vi "Function_Light.vi"(7 "Light Action":T1, 8 "Error in":errorcluster, 10 "Intensity":u8, 11 "Channel":u8) -> (0 "Error Out":errorcluster)   [LabVIEW 2013]
uses:
  Control/Control_Light.ctl
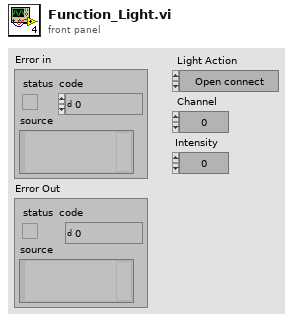
[diagram p1: front panel]
types:
  T1 = typedef "Control_Light.ctl" = enum16{"Open connect", "Close connect", "Open Light", "Set Value", "Close Light", "Idle"}
  T2 = enum16{"Standard", "Buffered", "CRLF", "Immediate"}
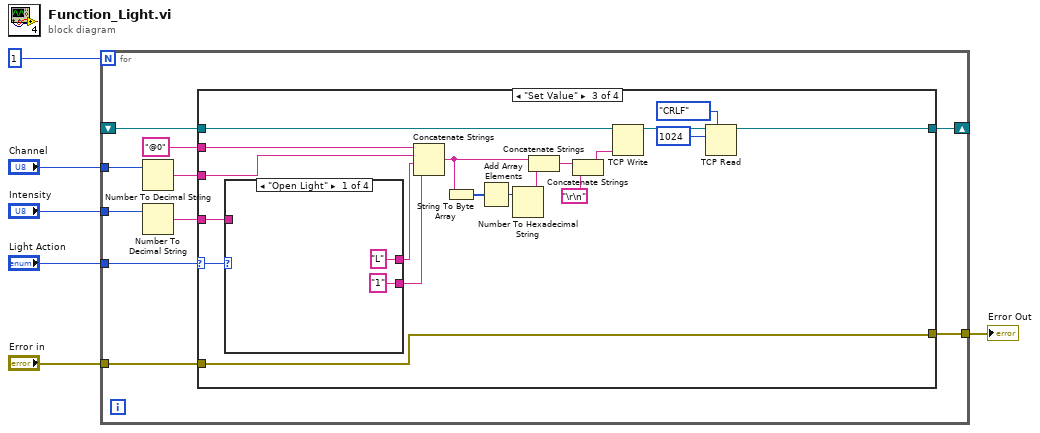
[diagram p0: block diagram]
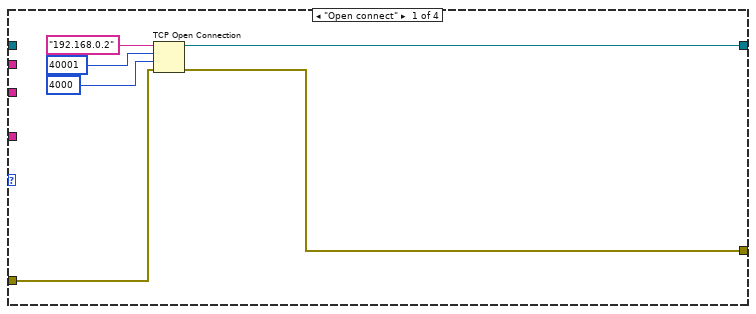
[diagram p2: hidden frame]
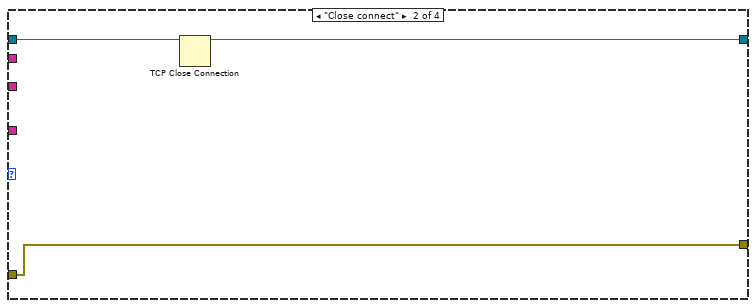
[diagram p3: hidden frame]
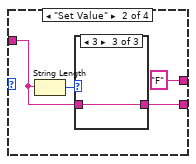
[diagram p4: hidden frame]
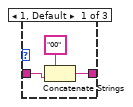
[diagram p5: hidden frame]
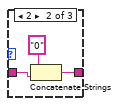
[diagram p6: hidden frame]
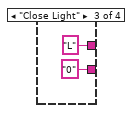
[diagram p7: hidden frame]
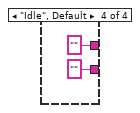
[diagram p8: hidden frame]
diagram:
  n1 = for {
    N: 1 -> [_]
    shift-right: [w15] -> _
    shift-left: _ -> [w12]
    tunnel: [w14] -> w5
    tunnel: "Error in" -> [w13]
    tunnel: "Channel" -> [w10]
    tunnel: "Intensity" -> [w8]
    tunnel: "Light Action" -> [w16]
    n2 = Number To Decimal String(number=w10) -> (decimal integer string=w9:string)  [unwired: 1 in]
    n3 = Number To Decimal String(number=w8) -> (decimal integer string=w7:string)  [unwired: 1 in]
    n4 = case shown="\"Set Value\"" w16 {
      selector: w16 -> [_ _ w26 _]
      tunnel: [w18 w24 w27 w63] -> w15
      tunnel: [w19 w23 w31 w62] -> w14
      tunnel: w13 -> [w17 w23 w31 w62]
      tunnel: w12 -> [_ w25 w35 w63]
      tunnel: "@0" ("string") -> [_ _ w33 _]
      tunnel: w9 -> [_ _ w34 _]
      tunnel: w7 -> [_ _ w32 _]
      frame "Open connect" {
        n5 = TCP Open Connection(address="192.168.0.2", remote port or service name=u16 40001, timeout ms (60000)=4000, error in (no error)=w17) -> (connection ID=w18:refnum<k5>, error out=w19:errorcluster)  [unwired: 1 in]
      }
      frame "Close connect" {
        n6 = TCP Close Connection(connection ID=w25) -> (connection ID out=w24:refnum<k5>)  [unwired: 2 in, 1 out]
      }
      frame "Set Value" {
        n7 = case shown="\"Open Light\"" w26 {
          tunnel: ["1" w49 "0" ""] -> w44
          tunnel: ["L" ("string") "F" ("string") "L" ("string") "" ("string")] -> w37
          tunnel: w32 -> [_ w48 _ _]
          frame "Open Light" {
          }
          frame "Set Value" {
            n8 = String Length(string=w48) -> (length=w47:i32)
            n9 = case shown="3" w47 {
              tunnel: [w53 w55 w57] -> w49
              tunnel: w48 -> [w52 w56 w57]
              frame 1, Default {
                n10 = Concatenate Strings("00" ("string"), w52) -> (w53:string)
              }
              frame 2 {
                n11 = Concatenate Strings("0" ("string"), w56) -> (w55:string)
              }
              frame 3 {
              }
            }
          }
          frame "Close Light" {
          }
          frame "Idle", Default {
          }
        }
        n12 = Concatenate Strings(w33, w34, w37, w44) -> (w38:string)
        n13 = String To Byte Array(string=w38) -> (unsigned byte array=w43:u8[])
        n14 = Add Array Elements(numeric array=w43) -> (sum=w42:u8)
        n15 = Number To Hexadecimal String(2:w42) -> (0:w41:string)  [unwired: 1 in]
        n16 = Concatenate Strings(w38, w41) -> (w39:string)
        n17 = Concatenate Strings(w39, "\r\n") -> (w36:string)
        n18 = TCP Write(connection ID=w35, data in=w36) -> (connection ID out=w28:refnum<k5>)  [unwired: 2 in, 2 out]
        n19 = TCP Read(connection ID=w28, bytes to read=1024, 7:T2."CRLF" ("mode (standard)")) -> (connection ID out=w27:refnum<k5>)  [unwired: 2 in, 2 out]
      }
      frame "Idle", Default {
      }
    }
  }
  "Error Out" <- w5
